vi "SimulateXYsignal.vi"(0 "Cluster":T1={"offset Xsignal [pN]"=20.0, "offset PX [nm]"=200.0, "offset PY [nm]"=100.0, "kBT"=4.1, "Noise lvl [pN]"=0.05, "Contour length [nm]"=2040.0, "Persistence length [nm]"=40.0, "step length [nm]"=10.0, "Total scan range [nm]"=2500.0, "trap height [nm]"=500.0}) -> (1 "XY Graph":cluster{dbl[], dbl[]}[](graph), 2 "XY Graph split":cluster{dbl[], dbl[]}[](graph))   [LabVIEW 2020, in "XYcenter.lvlib"]
uses:
  XYcenter.lvlib
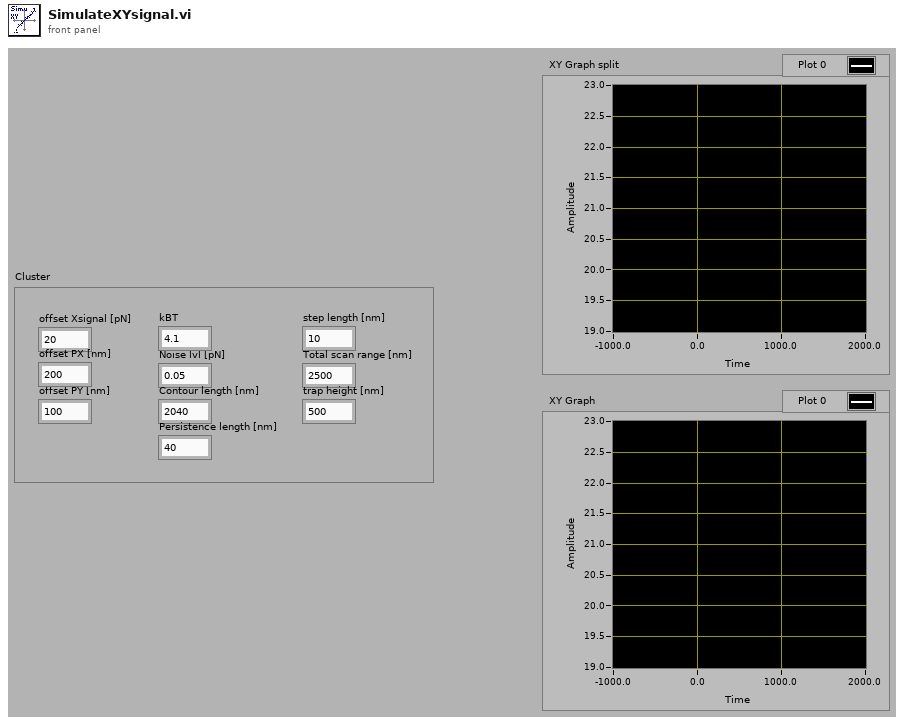
[diagram p1: front panel]
types:
  T1 = cluster{"offset Xsignal [pN]":dbl, "offset PX [nm]":dbl, "offset PY [nm]":dbl, "kBT":dbl, "Noise lvl [pN]":dbl, "Contour length [nm]":dbl, "Persistence length [nm]":dbl, "step length [nm]":dbl, "Total scan range [nm]":dbl, "trap height [nm]":dbl}
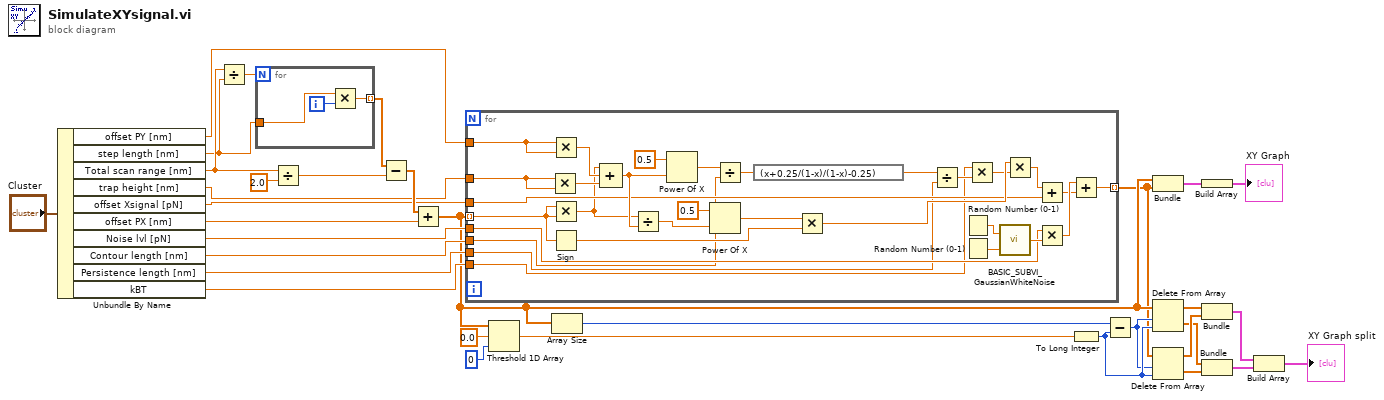
[diagram p0: block diagram]
diagram:
  n1 = Unbundle By Name("Cluster") -> ("offset PY [nm]"=w23:dbl, "step length [nm]"=w26:dbl, "Total scan range [nm]"=w27:dbl, "trap height [nm]"=w22:dbl, "offset Xsignal [pN]"=w18:dbl, "offset PX [nm]"=w25:dbl, "Noise lvl [pN]"=w24:dbl, "Contour length [nm]"=w19:dbl, "Persistence length [nm]"=w20:dbl, "kBT"=w21:dbl)
  n2 = Divide(x=w27, y=w26) -> (x/y=w33:dbl)
  n3 = for {
    N: w33 -> [_]
    tunnel: [w35] -> w31 mode=indexing
    tunnel: w26 -> [w34]
    i -> [w36]
    n4 = Multiply(x=w34, y=w36) -> (x*y=w35:dbl)
  }
  n5 = Divide(x=w27, y=2.0) -> (x/y=w30:dbl)
  n6 = Subtract(x=w31, y=w30) -> (x-y=w29:dbl[])
  n7 = Add(x=w29, y=w25) -> (x+y=w2:dbl[])
  n8 = for {
    tunnel: w2 -> [w54] mode=indexing
    tunnel: w23 -> [w66]
    tunnel: w22 -> [w65]
    tunnel: [w58] -> w1 mode=indexing
    tunnel: w18 -> [w49]
    tunnel: w24 -> [w41]
    tunnel: w21 -> [w40]
    tunnel: w20 -> [w39]
    tunnel: w19 -> [w38]
    n9 = Multiply(x=w65, y=w65) -> (x*y=w64:dbl)
    n10 = Multiply(x=w66, y=w66) -> (x*y=w63:dbl)
    n11 = Multiply(x=w54, y=w54) -> (x*y=w37:dbl)
    n12 = Sign(1:w54) -> (0:w53:dbl)
    n13 = Compound Arithmetic op=ADD(w37, w63, w64) -> (w59:dbl)
    n14 = Divide(x=w37, y=w59) -> (x/y=w62:dbl)
    n15 = Power Of X(1:w59, 2:0.5 ("y")) -> (0:w44:dbl)
    n16 = Power Of X(1:w62, 2:0.5 ("y")) -> (0:w52:dbl)
    n17 = Divide(x=w44, y=w38) -> (x/y=w43:dbl)
    n18 = expression code="(x+0.25/(1-x)/(1-x)-0.25)"(w43) -> (w46:dbl)
    n19 = Multiply(x=w52, y=w53) -> (x*y=w51:dbl)
    n20 = Divide(x=w46, y=w39) -> (x/y=w45:dbl)
    n21 = Random Number (0-1)() -> (number: 0 to 1=w56:dbl)
    n22 = Random Number (0-1)() -> (number: 0 to 1=w57:dbl)
    n23 = Multiply(x=w40, y=w45) -> (x*y=w42:dbl)
    n24 = call "BASIC_SUBVI_GaussianWhiteNoise.vi"("Rnd 2"=w57, "Rnd 1"=w56) -> ("NormalizedGaussianWhiteNoise"=w55:dbl)
    n25 = Multiply(x=w51, y=w42) -> (x*y=w48:dbl)
    n26 = Add(x=w48, y=w49) -> (x+y=w47:dbl)
    n27 = Multiply(x=w41, y=w55) -> (x*y=w50:dbl)
    n28 = Add(x=w50, y=w47) -> (x+y=w58:dbl)
  }
  n29 = Threshold 1D Array(1:0 ("start index (0)"), 2:0.0 ("threshold y"), 3:w2) -> (0:w15:dbl)
  n30 = Array Size(array=w2) -> (size(s)=w5:i32)
  n31 = To Long Integer(number=w15) -> (32bit integer=w14:i32)
  n32 = Subtract(x=w5, y=w14) -> (x-y=w13:i32)
  n33 = Bundle(w2, w1) -> (w4:cluster{dbl[], dbl[]})  [unwired: 1 in]
  n34 = Delete From Array(array=w2, length=w13, index=w14) -> (deleted portion=w6:dbl[], array with subset deleted=w11:dbl[])
  n35 = Delete From Array(array=w1, length=w13, index=w14) -> (deleted portion=w12:dbl[], array with subset deleted=w10:dbl[])
  n36 = Build Array(w4) -> (→"XY Graph":cluster{dbl[], dbl[]}[])
  n37 = Bundle(w11, w10) -> (w8:cluster{dbl[], dbl[]})  [unwired: 1 in]
  n38 = Bundle(w6, w12) -> (w9:cluster{dbl[], dbl[]})  [unwired: 1 in]
  n39 = Build Array(w8, w9) -> (→"XY Graph split":cluster{dbl[], dbl[]}[])
